vi "MB Read Multi Coils.vi"(8 "error in (no error)":errorcluster, 11 "Devices":T1) -> (0 "error out":errorcluster, 2 "Coils Name":string[](array[string]), 3 "coils":bool[](array[boolean]))   [LabVIEW 2021]
uses:
  <vilib>/NI/Modbus Library/API/Master/Modbus Master.lvclass
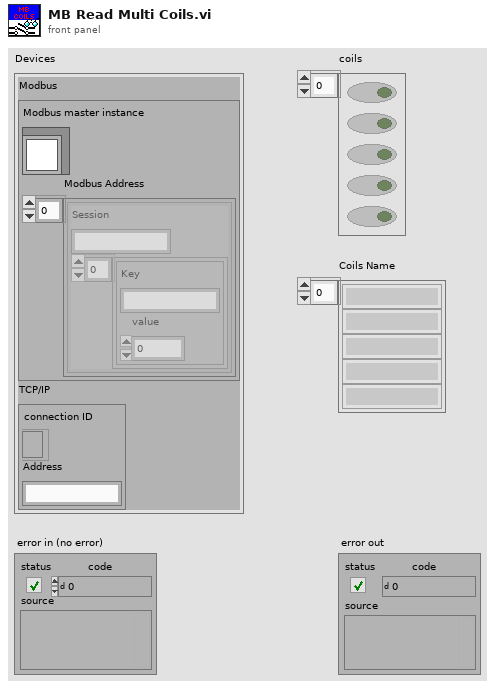
[diagram p1: front panel]
types:
  T1 = cluster{"Modbus":cluster{"Modbus master instance":refnum<class "Modbus Master.lvclass">, "Modbus Address":cluster{"Session":string, cluster{"Key":string, "value":u32}[]}[]}, "TCP/IP":cluster{"connection ID":refnum<k5>, "Address":string}}
  T2 = cluster{"Session":string, cluster{"Key":string, "value":u32}[]}[]
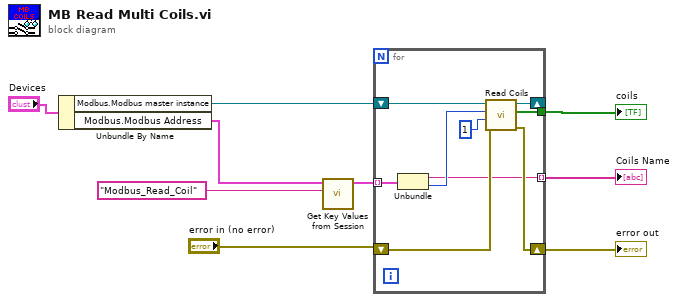
[diagram p0: block diagram]
diagram:
  n1 = Unbundle By Name("Devices") -> ("Modbus.Modbus master instance"=w9:refnum<class "Modbus Master.lvclass">, "Modbus.Modbus Address"=w5:T2)
  n2 = call "Get Key Values from Session.vi"("Session"="Modbus_Read_Coil", "Ini File"=w5) -> ("Keys Values in Session"=w4:cluster{"Key":string, "value":u32}[])  [unwired: 7 in, 2 out]
  n3 = for {
    tunnel: [w17] -> w7
    tunnel: w4 -> [w15] mode=indexing
    shift-right: [w13] -> _
    shift-left: w9 -> [w18]
    shift-right: [w11] -> w2
    shift-left: "error in (no error)" -> [w12]
    tunnel: [w10] -> w1 mode=indexing
    n4 = Unbundle(w15) -> ("Key"=w10:string, "value"=w14:u32)
    n5 = call-dynamic "Read Coils.vi"("error in"=w12, "number of inputs"=u16 1, "starting address"=w14, "Modbus master in"=w18) -> ("error out"=w11:errorcluster, "coils"=w17:bool[], "Modbus master out"=w13:refnum<class "Modbus Master.lvclass">)  [unwired: 5 in]
  }
  "coils" <- w7
  "error out" <- w2
  "Coils Name" <- w1
